vi "Plug Ins Main.vi"(8 "error in (no error)":errorcluster, 10 "Queue Name":string="Main") -> (0 "error out":errorcluster)   [LabVIEW 2011]
doc: "This is the main VI that searches for valid plug ins and then will call the appropriate one based on the user selecting it on a menu ring. The VI searches for Plug Ins every 250 milliseconds. The user may chose a different time frame or a different trigger for getting new plug ins and linking them to the application.\n\nAAL 9/09"
uses:
  Shared/QDMH Poly VIs/QDMH POLY Enqueue String.vi
  Shared/QDMH Poly VIs/QDMH POLY Enqueue Strings.vi
panel:
  out "Waveform Graph":waveform(dbl)(graph)
  in  "Waveform Selector":u16(ring) items=["Triangle Waveform", "Sine Waveform"]
  in  "Frequency":dbl=5.0
  in  "Amplitude":dbl=5.0
  out "Message Display":string
  in  "Cancel":bool
  in  "OK":bool
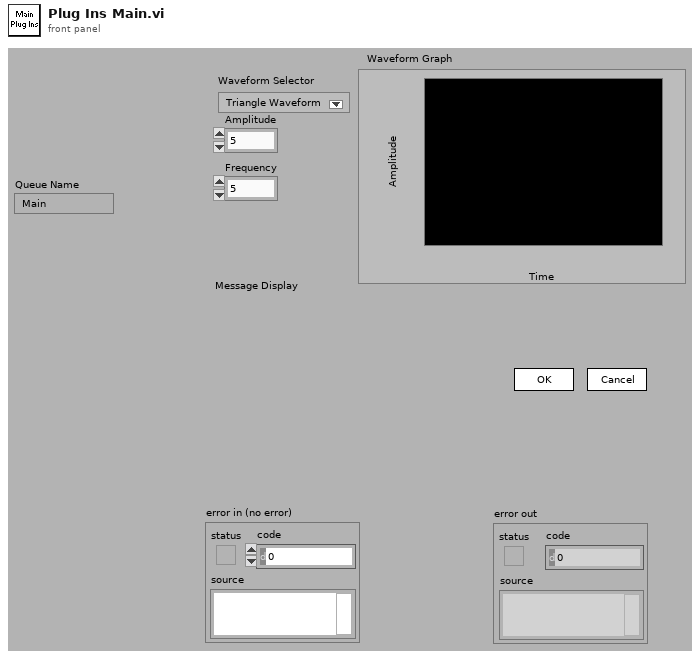
[diagram p1: front panel]
types:
  T1 = cluster{"Operator Name":string, "Current VI's Path":path, "Current VI's  Directory":path, "Queue Names":string[], "# VIs Launched":i32, "WFG Paths":path[], "Waveform Selection":i32, "Amplitude":dbl, "Frequency":dbl, "Plug Ins Directory":path, "Waveform":dbl[], "Signal out":waveform(dbl)}
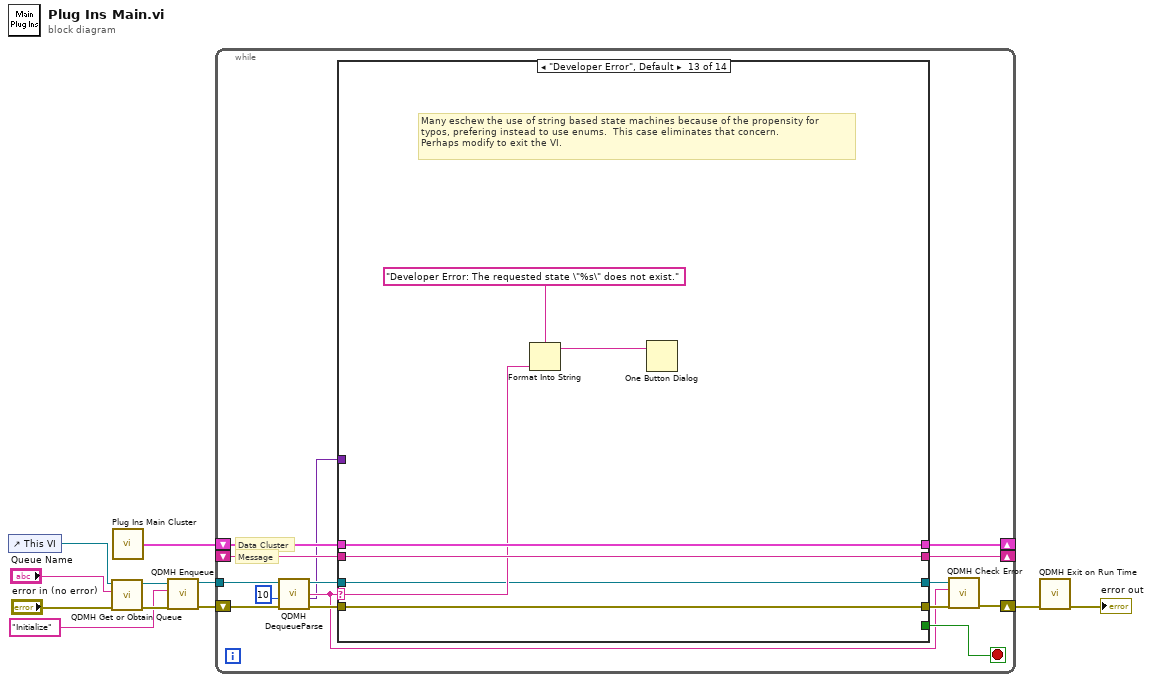
[diagram p0: block diagram]
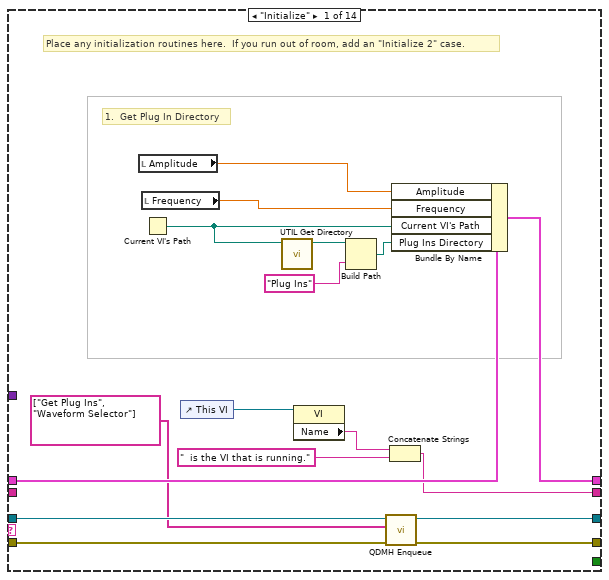
[diagram p2: hidden frame]
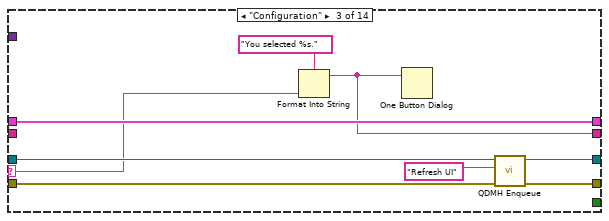
[diagram p4: hidden frame]
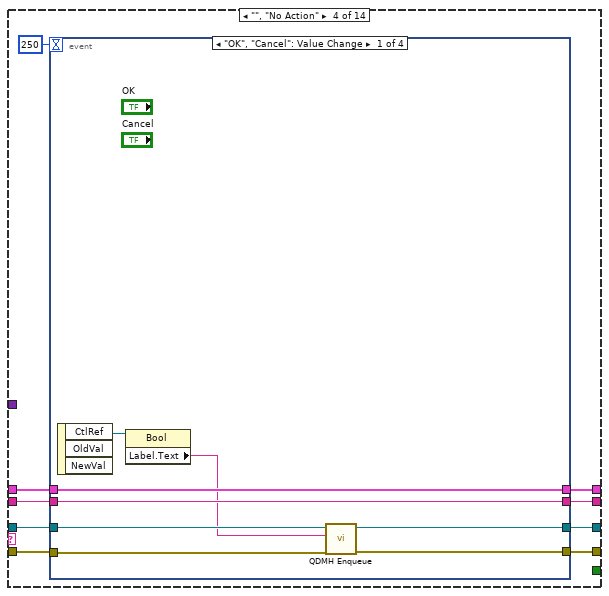
[diagram p5: hidden frame]
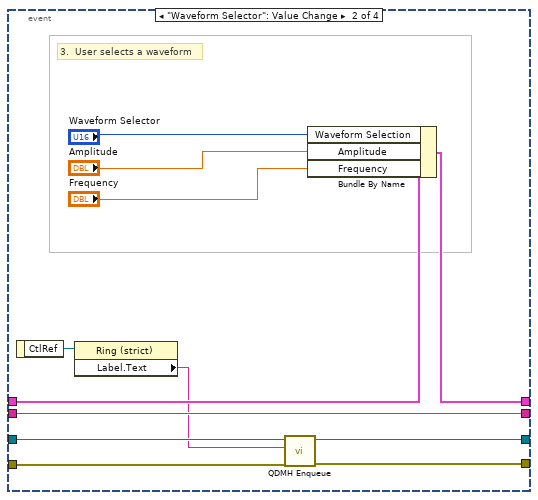
[diagram p6: hidden frame]
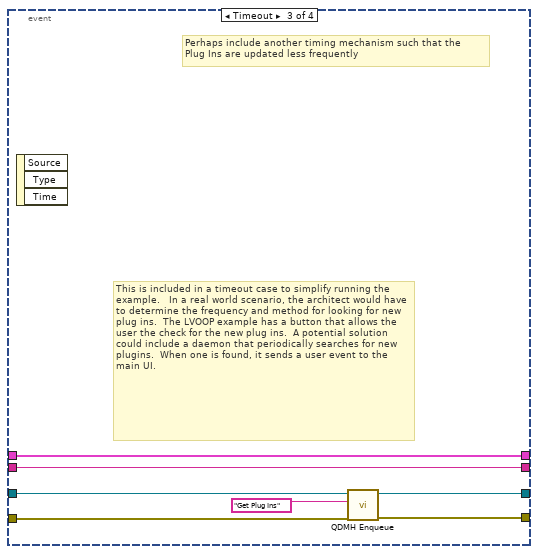
[diagram p7: hidden frame]
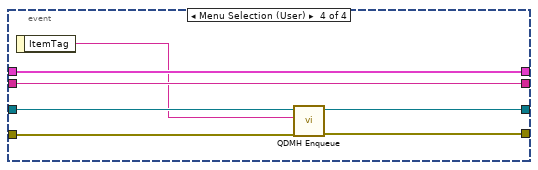
[diagram p8: hidden frame]
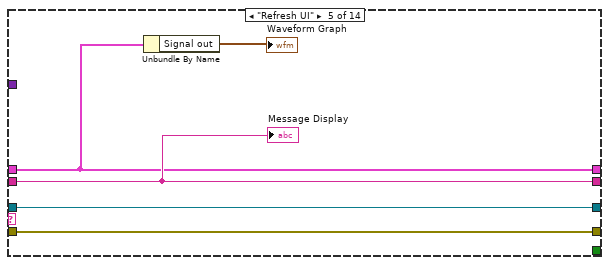
[diagram p9: hidden frame]
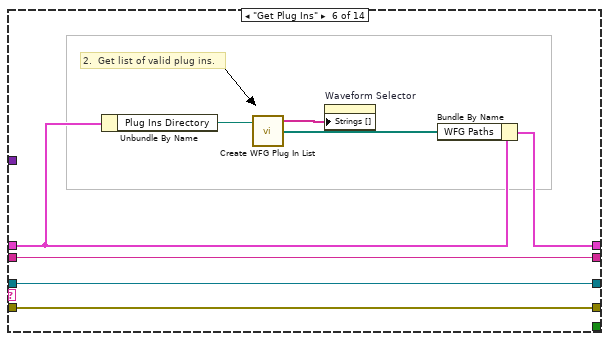
[diagram p10: hidden frame]
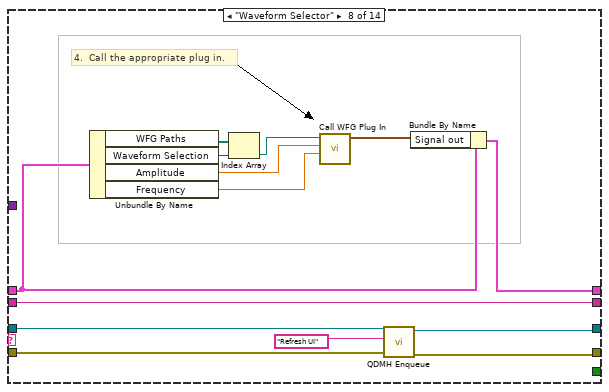
[diagram p12: hidden frame]
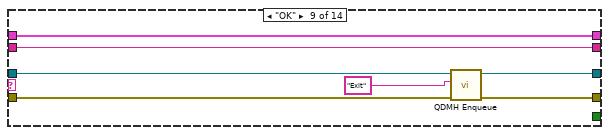
[diagram p13: hidden frame]
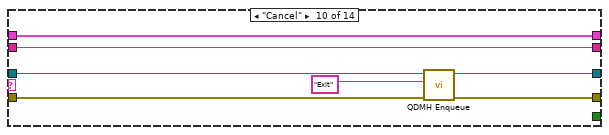
[diagram p14: hidden frame]
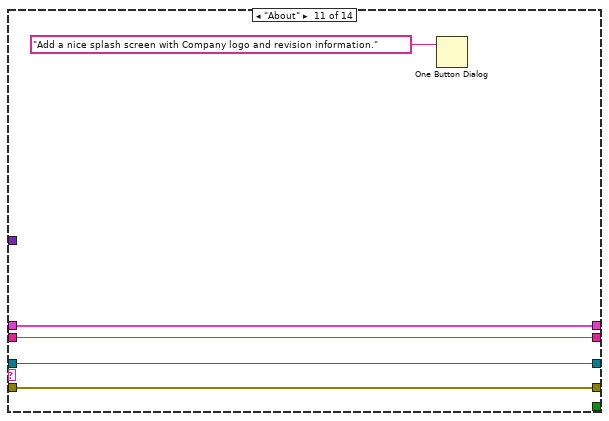
[diagram p15: hidden frame]
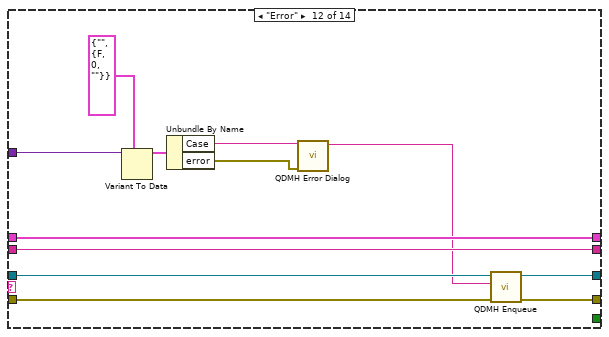
[diagram p16: hidden frame]
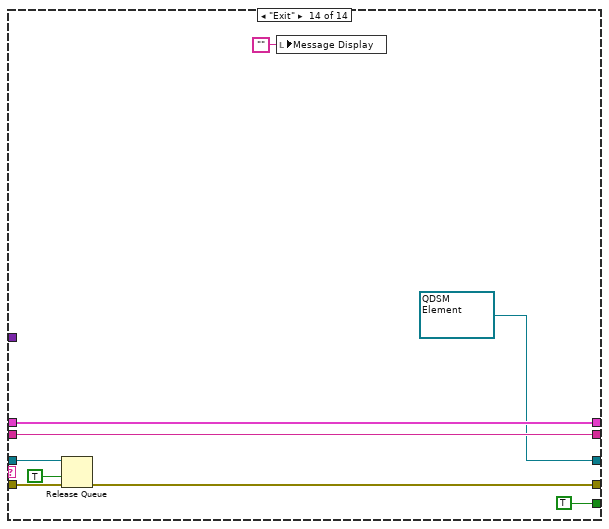
[diagram p17: hidden frame]
diagram:
  n1 = control-ref of="This VI"() -> (w3:refnum<vi>)
  n2 = call "QDMH Get or Obtain Queue.vi"("error in (no error)"="error in (no error)", "Queue Name"="Queue Name", "VI Refnum"=w3) -> ("error out"=w7:errorcluster, "queue out"=w10:refnum<queue>)  [unwired: 7 out]
  n3 = call "Plug Ins Main Cluster.vi"() -> ("Cluster"=w9:T1)
  n4 = call-poly "QDMH Enqueue.vi"("error in (no error)"=w7, "State"="Initialize" ("element"), "queue"=w10) -> ("error out"=w8:errorcluster, "queue out"=w11:refnum<queue>)  [unwired: 7 out]
  n5 = while {
    tunnel: w11 -> [w22]
    shift-left: w9 -> [w23]
    shift-right: [w24] -> _
    shift-left: _ -> [w25]
    shift-right: [w16] -> _
    shift-right: [w14] -> w5
    shift-left: w8 -> [w18]
    stop <- w26 stop-if-true
    # "Data Cluster"
    # "Message"
    n6 = call "QDMH DequeueParse.vi"("error in (no error)"=w18, "Timeout"=10 ("ms timeout (-1)"), "queue"=w22) -> ("error out"=w19:errorcluster, "Variant Data"=w12:variant, "State"=w13:string, "queue out"=w20:refnum<queue>)  [unwired: 5 out]
    n7 = case shown="\"Developer Error\", Default" w13 {
      selector: w13 -> [_ _ w52 _ _ _ _ _ _ _ _ _ w165 _]
      tunnel: w20 -> [w31 w44 w54 w65 w100 w105 w113 w121 w137 w144 w145 w159 w162 w174]
      tunnel: [_ _ _ _ _ _ _ _ _ _ _ _ _ TRUE] -> w26
      tunnel: [w40 w47 w53 w58 w104 w112 w116 w130 w136 w143 w149 w161 w168 w176] -> w16
      tunnel: w25 -> [_ w47 _ w59 w104 w112 w116 w130 w136 w143 w149 w161 w168 w176]
      tunnel: [w42 w46 w56 w60 w102 w106 w114 w122 w135 w142 w148 w160 w167 w171] -> w24
      tunnel: w23 -> [w43 w46 w56 w61 w102 w107 w114 w124 w135 w142 w148 w160 w167 w171]
      tunnel: w19 -> [w30 w45 w51 w64 w103 w111 w115 w120 w134 w141 w146 w158 w164 w173]
      tunnel: [w29 w45 w50 w63 w103 w111 w115 w119 w133 w140 w146 w157 w164 w170] -> w17
      tunnel: [w28 w44 w48 w57 w100 w105 w113 w118 w132 w139 w145 w156 w162 refnum<queue> refnum ("queue out")] -> w15
      tunnel: w12 -> [_ _ _ _ _ _ _ _ _ _ _ w151 _ _]
      frame "Initialize" {
        # "1.  Get Plug In Directory"
        # "Place any initialization routines here.  If you run out of room, add an \"Initialize 2\" case."
        n8 = local read "Amplitude"() -> (w33:dbl)
        n9 = local read "Frequency"() -> (w32:dbl)
        n10 = Current VI's Path() -> (path=w35:path)
        n11 = control-ref of="This VI"() -> (w39:refnum<vi>)
        n12 = call "UTIL Get Directory.vi"("Path In"=w35) -> ("Directory Out"=w36:path)  [unwired: 1 in, 9 out]
        n13 = property class="VI"(reference=w39) -> ("Name"=w38:string)  [unwired: 1 in, 2 out]
        n14 = Build Path(base path=w36, name or relative path="Plug Ins") -> (appended path=w34:path)
        n15 = call-poly "QDMH Enqueue.vi"("error in (no error)"=w30, "States"=string[] ["Get Plug Ins", "Waveform Selector"], "queue"=w31) -> ("error out"=w29:errorcluster, "queue out"=w28:refnum<queue>)  [unwired: 7 out]
        n16 = Concatenate Strings(w38, "  is the VI that is running." ("string")) -> (w40:string)
        n17 = Bundle By Name(cluster=w43, "Amplitude"=w33, "Frequency"=w32, "Current VI's Path"=w35, "Plug Ins Directory"=w34) -> (w42:T1)
      }
      frame "Re-Initialize" {
        # "This case includes initialization functionality that may need to run again during the course of the VI"
      }
      frame "Configuration" {
        n18 = Format Into String(format string="You selected %s." ("Format String"), w52) -> (resulting string=w53:string)  [unwired: 2 in, 1 out]
        n19 = One Button Dialog(message=w53) -> ()  [unwired: 2 out]
        n20 = call-poly "QDMH Enqueue.vi"("error in (no error)"=w51, "State"="Refresh UI" ("New State"), "queue"=w54) -> ("error out"=w50:errorcluster, "queue out"=w48:refnum<queue>)  [unwired: 7 out]
      }
      frame "", "No Action" {
        n21 = event shown="[0] \"OK\", \"Cancel\": Value Change" {
          selector: _ -> [_ _ _ _]
          dyn-events: _ -> [_ _ _ _]
          timeout: 250 -> [_ _ _ _]
          tunnel: w65 -> [w72 w85 w88 w99]
          tunnel: [w71 w84 w89 w97] -> w63
          tunnel: w64 -> [w70 w83 w90 w98]
          tunnel: w61 -> [w68 w81 w92 w96]
          tunnel: [w68 w80 w92 w96] -> w60
          tunnel: w59 -> [w69 w82 w91 w95]
          tunnel: [w69 w82 w91 w95] -> w58
          tunnel: [w66 w74 w87 w93] -> w57
          event "OK", "Cancel": Value Change {
            n22 = event-data() -> ("CtlRef"=w73:refnum<vi>)  [unwired: 3 out]
            n23 = property class="Bool"(reference=w73) -> ("Label.Text"=w67:string)  [unwired: 1 in, 2 out]
            n24 = call-poly "QDMH Enqueue.vi"("error in (no error)"=w70, "State"=w67, "queue"=w72) -> ("error out"=w71:errorcluster, "queue out"=w66:refnum<queue>)  [unwired: 7 out]
          }
          event "Waveform Selector": Value Change {
            # "3.  User selects a waveform"
            n25 = event-data() -> ("CtlRef"=w78:refnum<vi>)  [unwired: 1 out]
            n26 = property class="Ring (strict)"(reference=w78) -> ("Label.Text"=w75:string)  [unwired: 1 in, 2 out]
            n27 = call-poly "QDMH Enqueue.vi"("error in (no error)"=w83, "State"=w75, "queue"=w85) -> ("error out"=w84:errorcluster, "queue out"=w74:refnum<queue>)  [unwired: 7 out]
            n28 = Bundle By Name(cluster=w81, "Waveform Selection"="Waveform Selector", "Amplitude"="Amplitude", "Frequency"="Frequency") -> (w80:T1)
          }
          event Timeout {
            # "This is included in a timeout case to simplify running the example.   In a real world scenario, the architect would have to determine the frequency and method for looking for new plug ins.  The LVOOP example has a button that allows the user the check for the new plug ins.  A potential solution could include a daemon that periodically searches for new plugins.  When one is found, it sends a user event to the main UI."
            # "Perhaps include another timing mechanism such that the\nPlug Ins are updated less frequently"
            n29 = event-data() -> ()  [unwired: 4 out]
            n30 = call-poly "QDMH Enqueue.vi"("error in (no error)"=w90, "State"="Get Plug Ins" ("New State"), "queue"=w88) -> ("error out"=w89:errorcluster, "queue out"=w87:refnum<queue>)  [unwired: 7 out]
          }
          event Menu Selection (User) {
            n31 = event-data() -> ("ItemTag"=w94:string)  [unwired: 1 out]
            n32 = call-poly "QDMH Enqueue.vi"("error in (no error)"=w98, "State"=w94, "queue"=w99) -> ("error out"=w97:errorcluster, "queue out"=w93:refnum<queue>)  [unwired: 7 out]
          }
        }
      }
      frame "Refresh UI" {
        n33 = Unbundle By Name(w102) -> ("Signal out"=→"Waveform Graph":waveform(dbl))
        "Message Display" <- w104
      }
      frame "Get Plug Ins" {
        # "2.  Get list of valid plug ins."
        n34 = Unbundle By Name(w107) -> ("Plug Ins Directory"=w110:path)
        n35 = call "Create WFG Plug In List.vi"("path"=w110) -> ("menu names"=w109:string[], "VI paths"=w108:path[])  [unwired: 2 out]
        n36 = property on="Waveform Selector" class="Ring (strict)"("Strings []"=w109) -> ()  [unwired: 2 in, 2 out]
        n37 = Bundle By Name(cluster=w107, "WFG Paths"=w108) -> (w106:T1)
      }
      frame "<Add States As Needed>" {
        # "Duplicate this state for any additional states that you add."
      }
      frame "Waveform Selector" {
        # "4.  Call the appropriate plug in."
        n38 = Unbundle By Name(w124) -> ("WFG Paths"=w129:path[], "Waveform Selection"=w128:i32, "Amplitude"=w126:dbl, "Frequency"=w125:dbl)
        n39 = Index Array(array=w129, index=w128) -> (element=w127:path)
        n40 = call "Call WFG Plug In.vi"("Frequency"=w125, "Amplitude"=w126, "Plug-in VI Path"=w127) -> ("Signal out"=w123:waveform(dbl))  [unwired: 1 in, 7 out]
        n41 = call-poly "QDMH Enqueue.vi"("error in (no error)"=w120, "State"="Refresh UI" ("New State"), "queue"=w121) -> ("error out"=w119:errorcluster, "queue out"=w118:refnum<queue>)  [unwired: 7 out]
        n42 = Bundle By Name(cluster=w124, "Signal out"=w123) -> (w122:T1)
      }
      frame "OK" {
        n43 = call-poly "QDMH Enqueue.vi"("error in (no error)"=w134, "State"="Exit" ("New State"), "queue"=w137) -> ("error out"=w133:errorcluster, "queue out"=w132:refnum<queue>)  [unwired: 7 out]
      }
      frame "Cancel" {
        n44 = call-poly "QDMH Enqueue.vi"("error in (no error)"=w141, "State"="Exit" ("New State"), "queue"=w144) -> ("error out"=w140:errorcluster, "queue out"=w139:refnum<queue>)  [unwired: 7 out]
      }
      frame "About" {
        n45 = One Button Dialog(message="Add a nice splash screen with Company logo and revision information.") -> ()  [unwired: 2 out]
      }
      frame "Error" {
        n46 = Variant To Data(type=cluster{"Case":string, "error":errorcluster} {"Case"="", "error"={"status"=FALSE, "code"=0, "source"=""}} ("QDSM Element"), Variant=w151) -> (data=w153:cluster{"Case":string, "error":errorcluster})  [unwired: 1 in, 1 out]
        n47 = Unbundle By Name(w153) -> ("Case"=w154:string, "error"=w155:errorcluster)
        n48 = call "QDMH Error Dialog.vi"("error"=w155, "Case Error Occured"=w154) -> ("Case to Execute"=w150:string)  [unwired: 9 out]
        n49 = call-poly "QDMH Enqueue.vi"("error in (no error)"=w158, "State"=w150, "queue"=w159) -> ("error out"=w157:errorcluster, "queue out"=w156:refnum<queue>)  [unwired: 7 out]
      }
      frame "Developer Error", Default {
        # "Many eschew the use of string based state machines because of the propensity for\ntypos, prefering instead to use enums.  This case eliminates that concern.\nPerhaps modify to exit the VI."
        n50 = Format Into String(format string="Developer Error: The requested state \"%s\" does not exist." ("message"), w165) -> (resulting string=w163:string)  [unwired: 2 in, 1 out]
        n51 = One Button Dialog(message=w163) -> ()  [unwired: 2 out]
      }
      frame "Exit" {
        n52 = Release Queue(queue=w174, force destroy? (F)=TRUE, error in (no error)=w173) -> (error out=w170:errorcluster)  [unwired: 2 out]
        n53 = local write "Message Display"("") -> ()
      }
    }
    n54 = call "QDMH Check Error.vi"("error in (no error)"=w17, "Case"=w13, "queue"=w15) -> ("error out"=w14:errorcluster)  [unwired: 1 in, 7 out]
  }
  n55 = call "QDMH Exit on Run Time.vi"("error in (no error)"=w5) -> ("error out"=→"error out":errorcluster)  [unwired: 10 in]
